vi "open_im.vi"() -> ()   [LabVIEW 2020]
uses:
  <vilib>/wsapi/NI_WebServices.lvlib
panel:
  out "Array":dbl[](array[numeric])
  in  "im path":path=path "C:/Users/sindh/Desktop/LV CV/off1.png"
  out "String":string="[-11.74837723   9.80487245]"
  out "error out":errorcluster
  in  "error in (no error)":errorcluster
  in  "stop":bool
  in  "Run PY":bool
  in  "python module path":path=path "C:/Users/sindh/Desktop/LV CV/py_cv.py"
  in  "python function name":string="get_new_loc"
  in  "Python version":string="3.6"
  out "PY time":dbl=1718.0
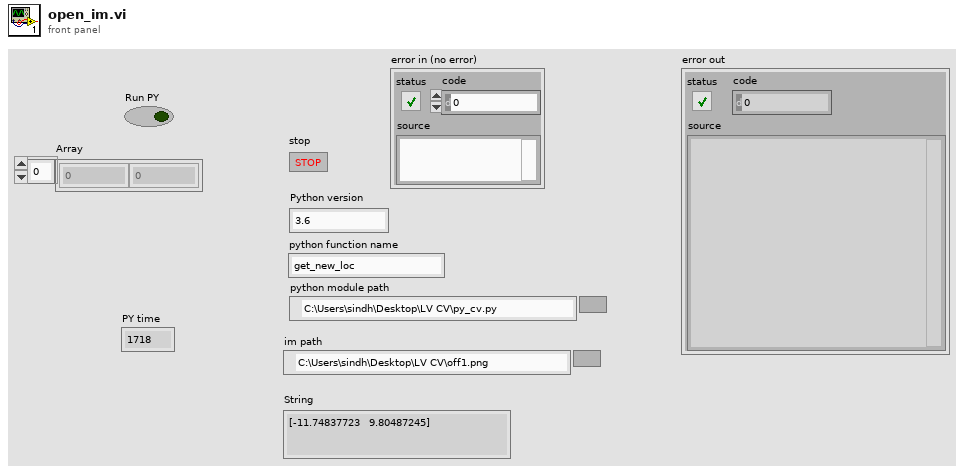
[diagram p1: front panel]
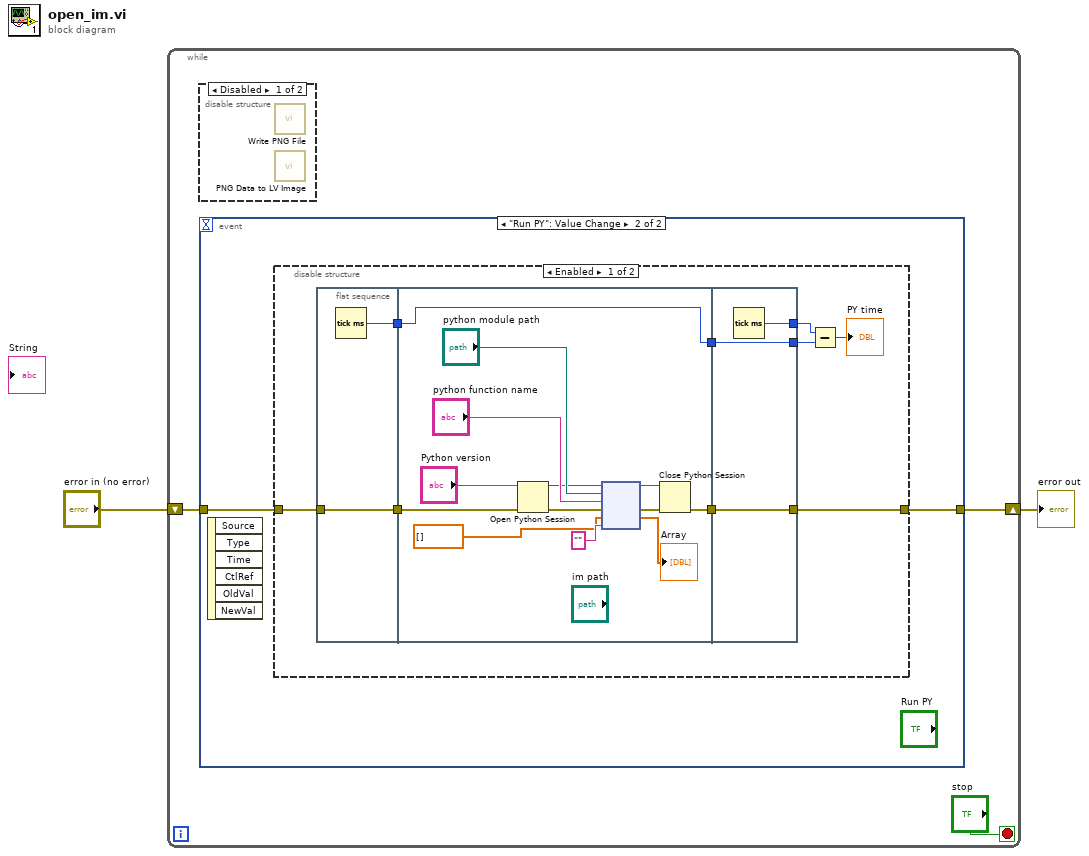
[diagram p0: block diagram]
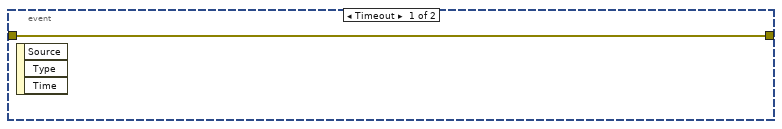
[diagram p3: hidden frame]
diagram:
  n1 = while {
    shift-right: [w4] -> w2
    shift-left: "error in (no error)" -> [w3]
    stop <- "stop" stop-if-true
    n2 = disable-structure shown="Disabled" {
      frame Disabled {
        n3 = call <vilib>:"Write PNG File.vi"() -> ()  [unwired: 10 in, 2 out]
        n4 = call <vilib>:"PNG Data to LV Image.vi"() -> ()  [unwired: 10 in, 2 out]
      }
      frame Enabled {
      }
    }
    n5 = event shown="[1] \"Run PY\": Value Change" {
      selector: _ -> [_ _]
      dyn-events: _ -> [_ _]
      timeout: _ -> [_ _]
      tunnel: w3 -> [w6 w8]
      tunnel: [w6 w7] -> w4
      event Timeout {
        n6 = event-data() -> ()  [unwired: 1 in, 3 out]
      }
      event "Run PY": Value Change {
        n7 = event-data() -> ()  [unwired: 1 in, 6 out]
        n8 = disable-structure shown="Enabled" {
          disable-tunnel: w8 -> [w13 _]
          disable-tunnel: [w12 _] -> w7
          frame Enabled {
            n9 = flat-sequence {
              tunnel: w13 -> [w19]
              tunnel: [w19] -> w17
              tunnel: [w18] -> w16
              tunnel: w17 -> [w27]
              tunnel: [w24] -> w15
              tunnel: [w23] -> w14
              tunnel: w16 -> [w23]
              tunnel: [w35] -> w12
              tunnel: w15 -> [w35]
              tunnel: [w34] -> w11
              tunnel: [w33] -> w10
              tunnel: w14 -> [w33]
              frame #0 {
                n10 = Tick Count (ms)() -> (millisecond timer value=w18:u32)
              }
              frame #1 {
                n11 = Open Python Session(python version="Python version", 3:w27) -> (session out=w29:refnum<k35>, error out=w26:errorcluster)  [unwired: 1 in]
                n12 = node(w29, "python module path", "python function name", w26, dbl[] [], "") -> (w30:refnum<k35>, w25:errorcluster, →"Array":dbl[])  [unwired: 1 in, 2 out]
                n13 = Close Python Session(session in=w30, error in=w25) -> (11:w24:errorcluster)
              }
              frame #2 {
                n14 = Tick Count (ms)() -> (millisecond timer value=w34:u32)
              }
            }
            n15 = Subtract(x=w11, y=w10) -> (x-y=→"PY time":u32)
          }
          frame Disabled {
          }
        }
      }
    }
  }
  "error out" <- w2
